vi "MoveLetter.vi"(8 "error in (no error)":errorcluster, 9 "Engine in":refnum<class "Engine.lvclass">, 11 "Highscore in":refnum<class "HighscoreDialog.lvclass">) -> (0 "error out":errorcluster, 1 "Engine out":refnum<class "Engine.lvclass">, 3 "Highscore out":refnum<class "HighscoreDialog.lvclass">)   [LabVIEW 2019, in "RT_Game.lvlib" / "HighscoreDialog.lvclass"]
uses:
  HighscoreDialog.lvclass
  Engine/Engine.lvclass
  HighscoreDialog.lvclass/HighscoreDialog.ctl
  Engine/Engine.lvclass/Engine.ctl
  Engine/Globals.vi
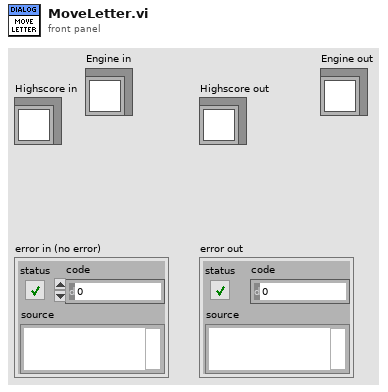
[diagram p1: front panel]
types:
  T1 = typedef "RT_Game.lvlib/Engine.lvclass/Controls.ctl" = cluster{"Controls_1":T2, "Controls_2":cluster{"DirectionX":i8, "DirectionY":i8, "Button1":bool, "Button2":bool}, "SystemButton":bool}
  T2 = typedef "RT_Game.lvlib/Engine.lvclass/ControlPlayer.ctl" = cluster{"DirectionX":i8, "DirectionY":i8, "Button1":bool, "Button2":bool}
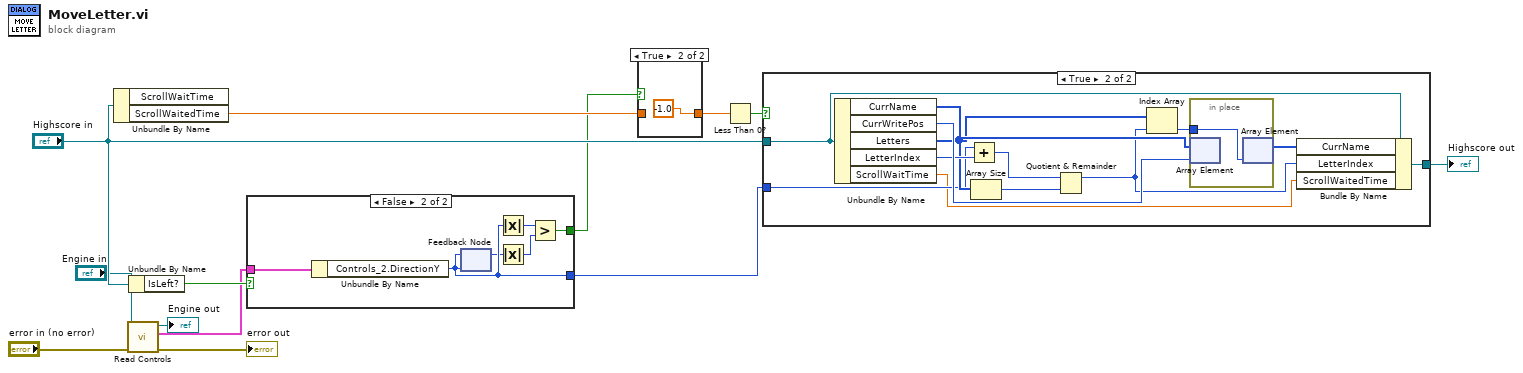
[diagram p0: block diagram]
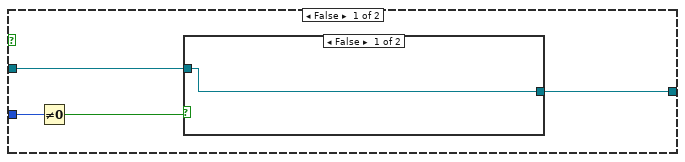
[diagram p3: hidden frame]
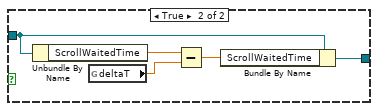
[diagram p4: hidden frame]
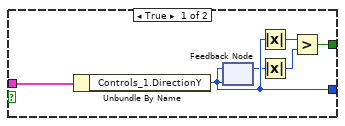
[diagram p5: hidden frame]
diagram:
  n1 = Unbundle By Name("Highscore in") -> ("ScrollWaitedTime"=w8:dbl)  [unwired: 1 out]
  n2 = call "Read Controls.vi"("error in (no error)"="error in (no error)", "Engine in"="Engine in") -> ("error out"=→"error out":errorcluster, "Controls"=w3:T1, "Engine out"=→"Engine out":refnum<class "Engine.lvclass">)  [unwired: 7 in]
  n3 = Unbundle By Name("Highscore in") -> ("IsLeft?"=w11:bool)
  n4 = case shown="False" w11 {
    tunnel: w3 -> [w19 w25]
    tunnel: [w18 w24] -> w10
    tunnel: [w15 w21] -> w5
    frame True {
      n5 = Unbundle By Name(w19) -> ("Controls_1.DirectionY"=w18:i8)
      n6 = feedback-in #1(w18) -> ()
      n7 = feedback #1(w18) -> (w16:i8)
      n8 = Absolute Value(x=w18) -> (abs(x)=w17:i8)
      n9 = Absolute Value(x=w16) -> (abs(x)=w14:i8)
      n10 = Greater?(x=w17, y=w14) -> (0:w15:bool)
    }
    frame False {
      n11 = Unbundle By Name(w25) -> ("Controls_2.DirectionY"=w24:i8)
      n12 = feedback-in #2(w24) -> ()
      n13 = feedback #2(w24) -> (w22:i8)
      n14 = Absolute Value(x=w24) -> (abs(x)=w23:i8)
      n15 = Absolute Value(x=w22) -> (abs(x)=w20:i8)
      n16 = Greater?(x=w23, y=w20) -> (0:w21:bool)
    }
  }
  n17 = case shown="True" w5 {
    tunnel: w8 -> [w26 _]
    tunnel: [w26 -1.0] -> w6
    frame False {
    }
    frame True {
    }
  }
  n18 = Less Than 0?(x=w6) -> (x < 0?=w7:bool)
  n19 = case shown="True" w7 {
    tunnel: [w31 w50] -> w13
    tunnel: "Highscore in" -> [w30 w49]
    tunnel: w10 -> [w29 w39]
    frame False {
      n20 = Not Equal To 0?(x=w29) -> (x != 0?=w28:bool)
      n21 = case shown="False" w28 {
        tunnel: [w32 w37] -> w31
        tunnel: w30 -> [w32 w36]
        frame False {
        }
        frame True {
          n22 = Unbundle By Name(w36) -> ("ScrollWaitedTime"=w35:dbl)
          n23 = global read "Globals.vi" "deltaT"() -> (w33:dbl)
          n24 = Subtract(x=w35, y=w33) -> (x-y=w34:dbl)
          n25 = Bundle By Name(cluster=w36, "ScrollWaitedTime"=w34) -> (w37:refnum<class "HighscoreDialog.lvclass">)
        }
      }
    }
    frame True {
      n26 = Unbundle By Name(w49) -> ("CurrName"=w48:u8[], "CurrWritePos"=w47:i16, "Letters"=w43:u8[], "LetterIndex"=w45:i16, "ScrollWaitTime"=w38:dbl)
      n27 = Add(x=w39, y=w45) -> (x+y=w44:i16)
      n28 = Array Size(array=w43) -> (size(s)=w42:i32)
      n29 = Quotient & Remainder(x=w44, y=w42) -> (x-y*floor(x/y)=w41:i32)  [unwired: 1 out]
      n30 = Index Array(array=w43, index=w41) -> (element=w40:u8)
      n31 = in-place {
        in-place-border: w40 -> [w51]
        n32 = in-place-array #3(w48, w47) -> ()  [unwired: 1 out]
        n33 = in-place-array #3(w51) -> (w46:u8[])  [unwired: 1 out]
      }
      n34 = Bundle By Name(cluster=w49, "CurrName"=w46, "LetterIndex"=w41, "ScrollWaitedTime"=w38) -> (w50:refnum<class "HighscoreDialog.lvclass">)
    }
  }
  "Highscore out" <- w13
